vi "pl1000SetPulseWidth.vi"(8 "error in (no error)":errorcluster, 9 "cycle":u8, 10 "period":u16, 11 "pl1000 handle":i16) -> (0 "error out":errorcluster, 3 "pl1000 handle out":i16)   [LabVIEW 2016, in "pl1000.lvlib"]
doc: "This function sets the pulse width of the PWM (pulse-width modulated) output. \n\nperiod: the required period of the PWM waveform in microseconds, from 100 to 1800\n\ncycle: the required duty cycle as a percentage from 0 to 100"
uses:
  pl1000.lvlib
  pl1000.dll
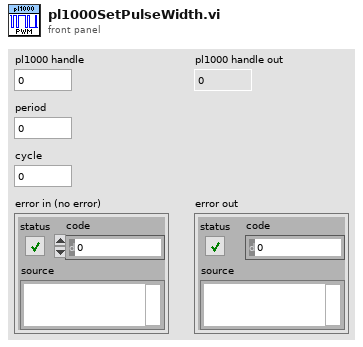
[diagram p1: front panel]
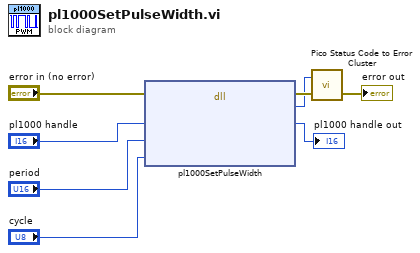
[diagram p0: block diagram]
diagram:
  n1 = dll-call lib="pl1000.dll" fn="pl1000SetPulseWidth"(error in="error in (no error)", "handle"="pl1000 handle", "period"="period", "cycle"="cycle") -> (error out=w6:errorcluster, "status"=w5:u32, "handle"=→"pl1000 handle out":i16)  [unwired: 4 in, 1 out]
  n2 = call "Pico Status Code to Error Cluster.vi"("error in"=w6, "PICO_STATUS"=w5) -> ("error out"=→"error out":errorcluster)  [unwired: 1 in]
